vi "Configure Reference Frequency.vi"(0 "VISA resource name":refnum<visa-resource-name>, 5 "Reference Source (0:Internal)":i32(ring) items=["Internal", "Auto"], 7 "Reference Frequency (0:10MHz)":i32(ring) items=["10 MHz", "13 MHz", "5 MHz"], 9 "Enable Reference Frequency (F:Disable)":bool, 11 "error in (no error)":errorcluster) -> (4 "VISA resource name out":refnum<visa-resource-name>, 15 "error out":errorcluster)   [LabVIEW 2020, in "Anritsu Signal Analyzer Series.lvlib"]
doc: "Selects the frequency reference signal source and Sets the reference signal frequency."
uses:
  Anritsu Signal Analyzer Series.lvlib
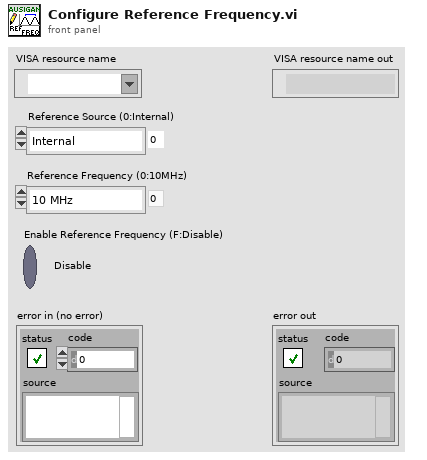
[diagram p1: front panel]
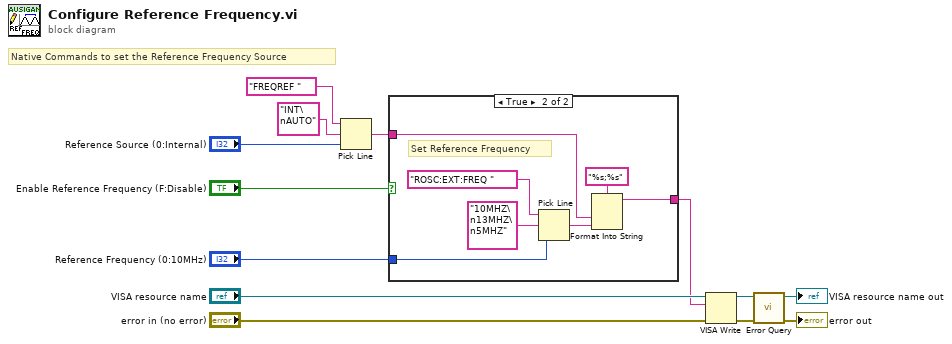
[diagram p0: block diagram]
diagram:
  # "Native Commands to set the Reference Frequency Source"
  n1 = Pick Line(string ("")="FREQREF " ("_CommandSet"), multi-line string="INT\nAUTO" ("_Case0"), line index="Reference Source (0:Internal)") -> (output string=w3:string)
  n2 = case shown="True" "Enable Reference Frequency (F:Disable)" {
    tunnel: "Reference Frequency (0:10MHz)" -> [_ w19]
    tunnel: w3 -> [w14 w17]
    tunnel: [w14 w15] -> w2
    frame False {
    }
    frame True {
      # "Set Reference Frequency"
      n3 = Pick Line(string ("")="ROSC:EXT:FREQ " ("_CommandSet"), multi-line string="10MHZ\n13MHZ\n5MHZ", line index=w19) -> (output string=w16:string)
      n4 = Format Into String(format string="%s;%s" ("形式文字列"), w17, w16) -> (resulting string=w15:string)  [unwired: 2 in, 1 out]
    }
  }
  n5 = VISA Write(VISA resource name="VISA resource name", write buffer=w2, error in (no error)="error in (no error)") -> (VISA resource name out=w9:refnum<visa-resource-name>, error out=w8:errorcluster)  [unwired: 1 out]
  n6 = call "Error Query.vi"("error in (no error)"=w8, "VISA resource name"=w9) -> ("error out"=→"error out":errorcluster, "VISA resource name out"=→"VISA resource name out":refnum<visa-resource-name>)  [unwired: 6 in, 2 out]
